vi "Change all structure ids.vi"() -> ()   [LabVIEW 2010]
uses:
  <vilib>/addons/database/NI_Database_API.lvlib
  <vilib>/addons/database/Connection.llb/DB Tools Open Connec (Path).vi
  <vilib>/addons/database/_DB Variant To Data/Database Variant To Data.xnode
  <vilib>/addons/database/Connection.llb/Conn Execute.vi
  <vilib>/addons/database/Recordset.llb/Rec Destroy - Connection.vi
panel:
  out "Numeric":i32
  in  "UDL":path=path "D:/Ab-initio/VASP Calcs/VASP DB.udl"
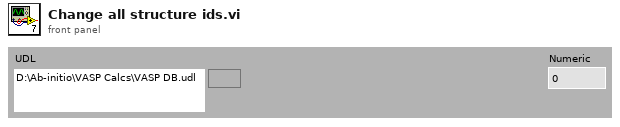
[diagram p1: front panel]
types:
  T1 = typedef "NI_Database_API.lvlib/Conn ObjectReference.ctl" = refnum<k1>
  T2 = cluster{"Structure Name":string, "Lattice vector a":dbl[], "Lattice vector b":dbl[], "Lattice vector c":dbl[], "Atoms Array":cluster{"Atom Name":string, "Positions (Direct)":dbl[][], "Positions (Cartesian)":dbl[][]}[], "# of atoms":i32}
  T3 = typedef "NI_Database_API.lvlib/Rec ObjectReference.ctl" = refnum<k1>
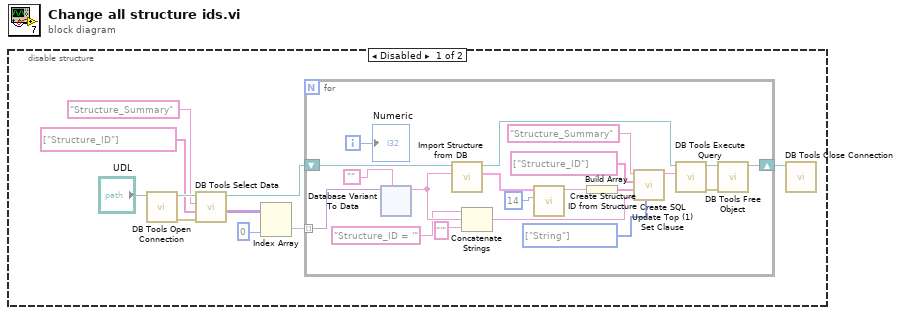
[diagram p0: block diagram]
diagram:
  n1 = disable-structure shown="Disabled" {
    frame Disabled {
      n2 = call-poly <vilib>:"DB Tools Open Connection.vi"("connection information"="UDL") -> ("error out"=w2:errorcluster, "connection reference"=w10:T1)  [unwired: 7 in]
      n3 = call <vilib>:"DB Tools Select Data.vi"("error in (no error)"=w2, "columns"=string[] ["Structure_ID"], "table"="Structure_Summary", "connection reference"=w10) -> ("data"=w6:variant[][], "connection reference out"=w8:T1)  [unwired: 2 in, 1 out]
      n4 = Index Array(array=w6, index (col)=0 ("disabled index (col)")) -> (element=w4:variant[])  [unwired: 1 in]
      n5 = for {
        shift-right: [w13] -> w7
        shift-left: w8 -> [w29]
        tunnel: w4 -> [w28] mode=indexing
        i -> [w11]
        w23 = enum16{"String", "Number", "Date-Time"}[] [enum."String"] items=["String", "Number", "Date-Time"] ("Data Types")
        n6 = xnode "Database Variant To Data"("database variant"=w28, "type"="") -> ("data"=w22:string)  [unwired: 1 in, 1 out]
        n7 = call "Import Structure from DB.vi"("Structure ID"=w22, "connection reference"=w29) -> ("Loaded Structure"=w30:T2, "connection reference out"=w15:T1)  [unwired: 7 in, 1 out]
        n8 = Concatenate Strings("Structure_ID = '" ("string"), w22, "'" ("string")) -> (w19:string)
        n9 = call "Create Structure ID from Structure.vi"("ID Length"=14, "Structure"=w30) -> ("Structure ID"=w25:string)  [unwired: 9 in]
        n10 = Build Array(w25) -> (w24:string[])
        n11 = call "Create SQL Update Top (1) Set Clause.vi"("Data Types"=w23, "Where Clause"=w19, "New Data (Strings)"=w24, "Column Headers"=string[] ["Structure_ID"], "Table to Update"="Structure_Summary") -> ("SET Statement"=w16:string)  [unwired: 6 in]
        n12 = call-poly <vilib>:"DB Tools Execute Query.vi"("SQL query"=w16, "connection reference"=w15) -> ("error out"=w12:errorcluster, "recordset reference"=w14:T3)  [unwired: 6 in]
        n13 = call-poly <vilib>:"DB Tools Free Object.vi"("error in (no error)"=w12, "recordset reference"=w14) -> ("connection reference"=w13:T1)  [unwired: 8 in, 1 out]
        "Numeric" <- w11
      }
      n14 = call <vilib>:"DB Tools Close Connection.vi"("connection reference"=w7) -> ()  [unwired: 6 in, 1 out]
    }
    frame Enabled {
    }
  }
